vi "SEARCH_VENDING MACHINE.vi"(8 "error in (no error)":errorcluster, 11 "USR":T1) -> (0 "error out":errorcluster, 2 "found?":bool, 3 "USR":T1)   [LabVIEW 2019, in "DB_VENDING MACHINE.lvlib"]
uses:
  DB_VENDING MACHINE.lvlib
  6 SEMESTRE/ADQUISICION_DATOS/BASE DE DATOS WEB/DB_LIBRARY/USR.ctl
  <vilib>/addons/database/_DB Variant To Data/Database Variant To Data.xnode
  <vilib>/addons/database/NI_Database_API.lvlib
  6 SEMESTRE/ADQUISICION_DATOS/BASE DE DATOS WEB/DB_LIBRARY/DB_LIBARY.lvlib
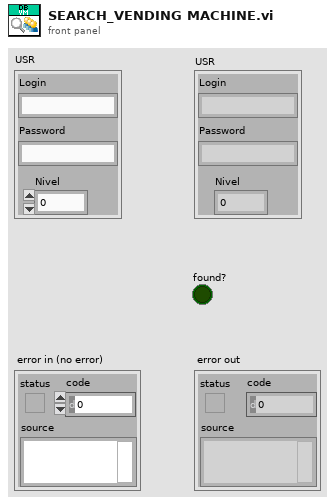
[diagram p1: front panel]
types:
  T1 = typedef "DB_LIBARY.lvlib/USR.ctl" = cluster{"Login":string, "Password":string, "Nivel":u8}
  T2 = typedef "NI_Database_API.lvlib/Conn ObjectReference.ctl" = refnum<k1>
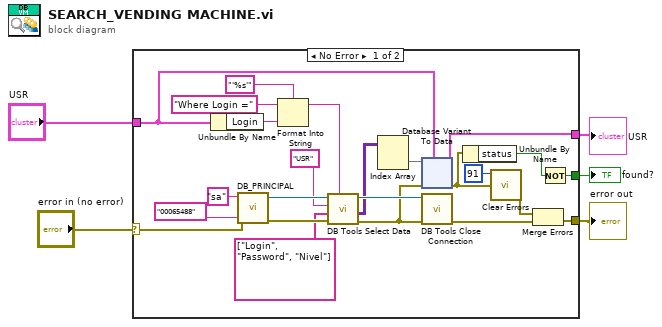
[diagram p0: block diagram]
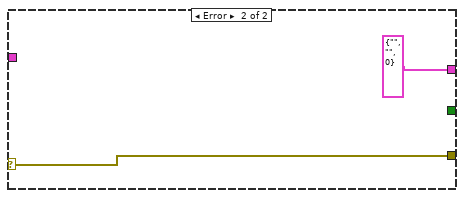
[diagram p2: hidden frame]
diagram:
  n1 = case shown="No Error" "error in (no error)" {
    selector: "error in (no error)" -> [w21 w128]
    tunnel: "USR" -> [w14 _]
    tunnel: [w7 w128] -> w4
    tunnel: [w13 T1 {"Login"="", "Password"="", "Nivel"=0} ("data")] -> w2
    tunnel: [w10 _] -> w1
    frame No Error {
      n2 = Unbundle By Name(w14) -> ("Login"=w19:string)
      n3 = call "DB_PRINCIPAL.vi"("error in (no error)"=w21, "password"="00065488", "userID"="sa") -> ("error out"=w28:errorcluster, "connection reference"=w29:T2)  [unwired: 7 in]
      n4 = Format Into String(format string="'%s'", initial string="Where Login =" ("condition"), w19) -> (resulting string=w17:string)  [unwired: 1 in, 1 out]
      n5 = call <vilib>:"DB Tools Select Data.vi"("condition"=w17, "error in (no error)"=w28, "columns"=string[] ["Login", "Password", "Nivel"], "table"="USR", "connection reference"=w29) -> ("error out"=w12:errorcluster, "data"=w16:variant[][], "connection reference out"=w27:T2)  [unwired: 1 in]
      n6 = Index Array(array=w16) -> (element=w15:variant[])  [unwired: 2 in]
      n7 = xnode "Database Variant To Data"("database variant"=w15, "error in (no error)"=w12, "type"=w14) -> ("data"=w13:T1, "error out"=w9:errorcluster)
      n8 = call <vilib>:"DB Tools Close Connection.vi"("error in (no error)"=w12, "connection reference"=w27) -> ("error out"=w22:errorcluster)  [unwired: 5 in]
      n9 = Unbundle By Name(w9) -> ("status"=w11:bool)
      n10 = call <vilib>:"Clear Errors.vi"("error in (no error)"=w9, "specific error code to clear (0: all)"=91) -> ("error out"=w6:errorcluster)  [unwired: 4 in, 1 out]
      n11 = Merge Errors(w6, w22) -> (w7:errorcluster)
      n12 = Not(x=w11) -> (.not. x?=w10:bool)
    }
    frame Error {
    }
  }
  "error out" <- w4
  "USR" <- w2
  "found?" <- w1
